vi "Finish.vi"   [LabVIEW 2017]
doc: "This VI is called just before exiting. It is expected to close I/O refnum, save collected data, etc."
uses:
  <vilib>/Rock Robotics/WPI/Utilities/WPI_GetSetVariantRefNum.vi
types:
  T1 = typedef "WPI_CompressorDevRef.ctl" = cluster{"DevStatus":errorcluster, "Pneumatics Control Module":u8}
  T2 = typedef "WPI_RobotDriveDevRef.ctl" = cluster{"DevStatus":errorcluster, "Motors[]":T3[], "Square Inputs":bool, "Max Output":dbl}
  T3 = typedef "WPI_MotorControlDeviceRef.ctl" = cluster{"DeviceStatus":errorcluster, "Type":T4, "PWM":cluster{"PWM Channel":T5, "DeadBand":T6}, "CAN":cluster{"Device Number":u8, "SetOutput VI Ref":variant, "GetOutput VI Ref":variant, "Enable VI Ref":variant, "Disable VI Ref":variant, "Data":variant}, "Invert":bool, "DIO PWM":cluster{"PWM \"Enable\" Channel":T5, "DIOChannel":T7, "PWM Rate":dbl}}
  T4 = typedef "WPI_MotorControlType.ctl" = enum16{"PWM", "CAN", "DIO PWM"}
  T5 = typedef "FPGA_DIOPWMChannel.ctl" = enum8{"PWM 0", "PWM 1", "PWM 2", "PWM 3", "PWM 4", "PWM 5", "PWM 6", "PWM 7", "PWM 8", "PWM 9", "PWM MXP 0", "PWM MXP 1", "PWM MXP 2", "PWM MXP 3", "PWM MXP 4", "PWM MXP 5", "PWM MXP 6", "PWM MXP 7", "PWM MXP 8", "PWM MXP 9", "Invalid"}
  T6 = typedef "WPI_PWMDeadband.ctl" = cluster{"Name":string, "maxPositivePwm":i32, "minPositivePwm":i32, "centerPwm":i32, "maxNegativePwm":i32, "minNegativePwm":i32, "angularRange":u16}
  T7 = typedef "FPGA_DIOChannel.ctl" = enum8{"DIO 0", "DIO 1", "DIO 2", "DIO 3", "DIO 4", "DIO 5", "DIO 6", "DIO 7", "DIO 8", "DIO 9", "DIO MXP 0", "DIO MXP 1", "DIO MXP 2", "DIO MXP 3", "DIO MXP 4", "DIO MXP 5", "DIO MXP 6", "DIO MXP 7", "DIO MXP 8", "DIO MXP 9", "DIO MXP 10", "DIO MXP 11", "DIO MXP 12", "DIO MXP 13", "DIO MXP 14", "DIO MXP 15", "SPI Port CS1", "SPI Port CS2", "SPI Port CS3", "SPI Port MISO", "SPI Port MOSI", "Invalid"}
  T8 = typedef "WPI_JoystickDevRef.ctl" = cluster{"Device":T9}
  T9 = typedef "WPI_JoystickDeviceEnum.ctl" = enum16{"USB 0", "USB 1", "USB 2", "USB 3", "USB 4", "USB 5"}
  T10 = typedef "WPI_GyroDevRef.ctl" = cluster{"DevStatus":errorcluster, "Analog Channel":T11, "Gain (VoltsPerDegree/Second)":dbl, "Gyro Type":enum16{"Analog", "XRS450"}, "Handle":i32, "SPI Bus":T12, "Device Found":bool, "Sample Rate":dbl, "Calibrate On Open":bool, "Offset":dbl}
  T11 = typedef "FPGA_AIChannel.ctl" = enum8{"AI 0", "AI 1", "AI 2", "AI 3", "AI MXP 0", "AI MXP 1", "AI MXP 2", "AI MXP 3", "Invalid"}
  T12 = typedef "spi_bus.ctl" = enum16{"SPI On-Board, CS0", "SPI On-Board, CS1", "SPI On-Board, CS2", "SPI On-Board, CS3", "SPI MXP", "Invalid"}
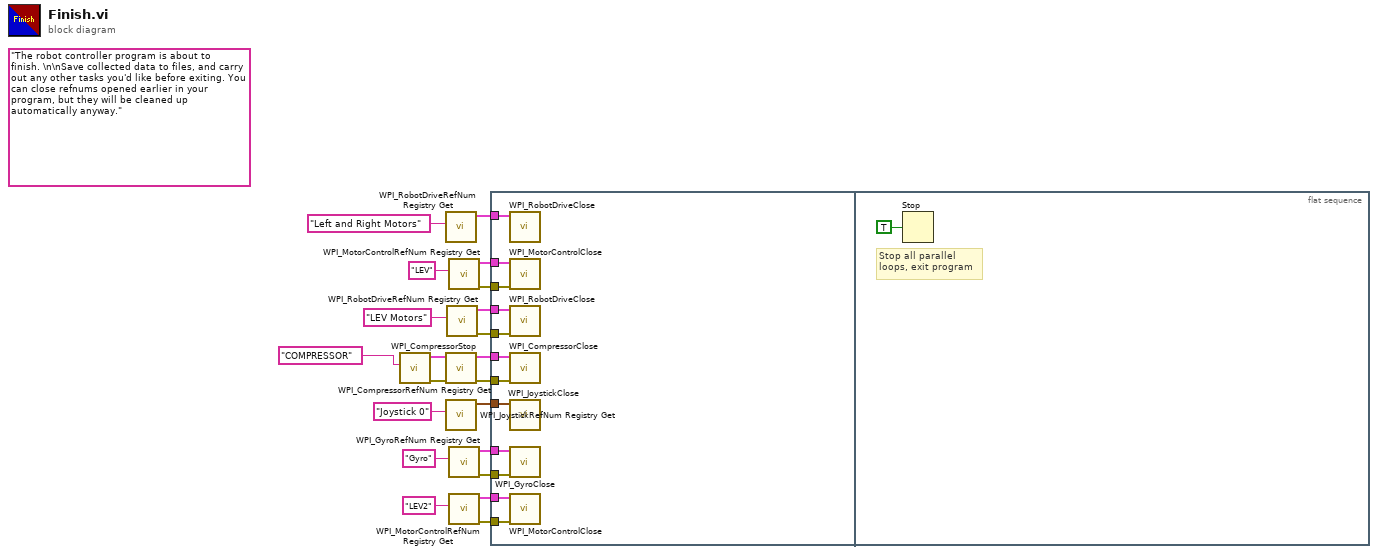
[diagram p0: block diagram]
diagram:
  (unwired) "The robot controller program is about to finish. \n\nSave collected data to files, and carry out any other tasks you'd like before exiting. You can close refnums opened earlier in your program, but they will be cleaned up automatically anyway."
  n1 = call <vilib>:"WPI_CompressorRefNum Registry Get.vi"("refnum name"="COMPRESSOR") -> ("error out"=w5:errorcluster, "CompressorDevRef"=w4:T1)  [unwired: 9 in]
  n2 = call <vilib>:"WPI_RobotDriveRefNum Registry Get.vi"("refnum name"="Left and Right Motors") -> ("RobotDriveDevRef"=w19:T2)  [unwired: 1 in, 9 out]
  n3 = call <vilib>:"WPI_CompressorStop.vi"("error in (no error)"=w5, "CompressorDevRef"=w4) -> ("error out"=w2:errorcluster, "CompressorDevRef"=w3:T1)  [unwired: 8 in]
  n4 = call <vilib>:"WPI_JoystickRefNum Registry Get.vi"("refnum name"="Joystick 0") -> ("JoystickDevRef"=w18:T8)  [unwired: 1 in, 9 out]
  n5 = call <vilib>:"WPI_RobotDriveRefNum Registry Get.vi"("refnum name"="LEV Motors") -> ("error out"=w10:errorcluster, "RobotDriveDevRef"=w11:T2)  [unwired: 9 in]
  n6 = call <vilib>:"WPI_MotorControlRefNum Registry Get.vi"("refnum name"="LEV") -> ("error out"=w15:errorcluster, "MotorControlDevRef"=w16:T3)  [unwired: 9 in]
  n7 = call <vilib>:"WPI_GyroRefNum Registry Get.vi"("refnum name"="Gyro") -> ("error out"=w6:errorcluster, "GyroDevRef"=w7:T10)  [unwired: 9 in]
  n8 = call <vilib>:"WPI_MotorControlRefNum Registry Get.vi"("refnum name"="LEV2") -> ("error out"=w14:errorcluster, "MotorControlDevRef"=w13:T3)  [unwired: 9 in]
  n9 = flat-sequence {
    tunnel: w19 -> [w33]
    tunnel: w18 -> [w32]
    tunnel: w16 -> [w31]
    tunnel: w15 -> [w30]
    tunnel: w13 -> [w28]
    tunnel: w14 -> [w29]
    tunnel: w11 -> [w27]
    tunnel: w10 -> [w26]
    tunnel: w7 -> [w25]
    tunnel: w6 -> [w24]
    tunnel: w3 -> [w23]
    tunnel: w2 -> [w22]
    frame #0 {
      n10 = call <vilib>:"WPI_RobotDriveClose.vi"("RobotDriveDevRef"=w33) -> ()  [unwired: 1 in, 10 out]
      n11 = call <vilib>:"WPI_MotorControlClose.vi"("error in"=w30, "MotorControlDevRef"=w31) -> ()  [unwired: 9 in, 1 out]
      n12 = call <vilib>:"WPI_RobotDriveClose.vi"("error in (no error)"=w26, "RobotDriveDevRef"=w27) -> ()  [unwired: 9 in, 1 out]
      n13 = call <vilib>:"WPI_CompressorClose.vi"("error in (no error)"=w22, "CompressorDevRef"=w23) -> ()  [unwired: 9 in, 1 out]
      n14 = call <vilib>:"WPI_JoystickClose.vi"("JoystickDevRef"=w32) -> ()  [unwired: 11 out]
      n15 = call <vilib>:"WPI_GyroClose.vi"("error in"=w24, "GyroDevRef"=w25) -> ()  [unwired: 9 in, 1 out]
      n16 = call <vilib>:"WPI_MotorControlClose.vi"("error in"=w29, "MotorControlDevRef"=w28) -> ()  [unwired: 9 in, 1 out]
    }
    frame #1 {
      # "Stop all parallel\nloops, exit program"
      n17 = Stop(stop? (T)=TRUE ("Quit")) -> ()
    }
  }
